vi "CLS.vi"(0 "System no.":i32=1 min=1 max=4 step=1, 5 "error in":errorcluster) -> (19 "error out":errorcluster)   [LabVIEW 2026]
doc: "Clears the controller display."
panel:
  # "Clears the controller display."
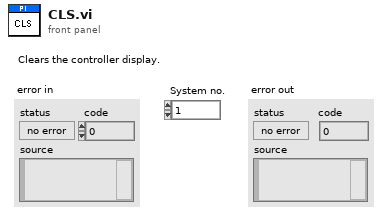
[diagram p1: front panel]
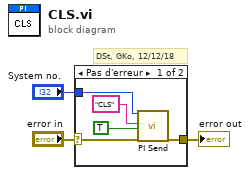
[diagram p0: block diagram]
diagram:
  # "DSt, GKo, 12/12/18"
  n1 = case shown="Pas d'erreur" "error in" {
    selector: "error in" -> [w6 w9]
    tunnel: "System no." -> [w8 _]
    tunnel: [w7 w9] -> w2
    frame No Error {
      n2 = call "PI Send.vi"("System no."=w8, "String to send"="CLS", "Attach termination char.?"=TRUE ("Attach Linefeed?"), "error in"=w6) -> ("error out"=w7:errorcluster)  [unwired: 2 in, 13 out]
    }
    frame Error {
    }
  }
  "error out" <- w2
